vi "Get settings chain.vi"(8 "error in (no error)":errorcluster, 11 "TemplateBase in":refnum<class "PockelCell.lvclass">) -> (0 "error out":errorcluster, 1 "class name":string[](array[string]), 2 "settings":variant[](array[variant]), 3 "TemplateBase out":refnum<class "PockelCell.lvclass">)   [LabVIEW 2012, in "PockelCell.lvclass"]
doc: "Returns an array of variants containing the settings clusters of each class in the inheritance chain (lowest child class first), together with an array of all class names in the inheritance chain.\n\nFor classes without settings cluster, the settings chain contains empty variants."
uses:
  PockelCell.lvclass
  <vilib>/Distrio/Murmex/Murmex/Murmex.lvclass
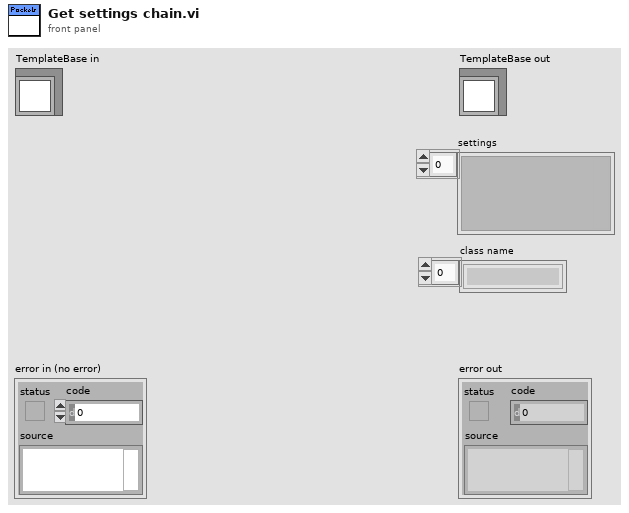
[diagram p1: front panel]
types:
  T1 = typedef "PockelCell.lvclass/settings_cluster.ctl" = cluster{"Samples per cycle":i32, "Number of cycles":i32, "Duty cycle (%)":dbl, "Analog Voltage\n":T2}
  T2 = typedef "PockelCell.lvclass/laser line PC.ctl" = dbl
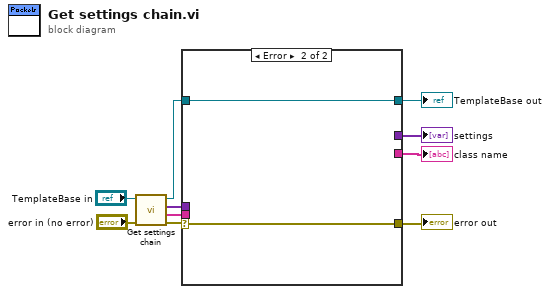
[diagram p0: block diagram]
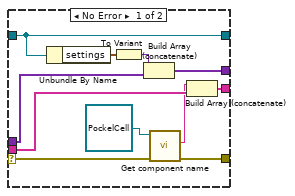
[diagram p2: hidden frame]
diagram:
  n1 = call-parent "Get settings chain.vi"("error in (no error)"="error in (no error)", "MurmexBase in"="TemplateBase in") -> ("error out"=w8:errorcluster, "class name"=w3:string[], "settings"=w4:variant[], "MurmexBase out"=w6:refnum<class "PockelCell.lvclass">)  [unwired: 6 in]
  n2 = case shown="Error" w8 {
    selector: w8 -> [w21 w22]
    tunnel: [w20 w22] -> w7
    tunnel: w6 -> [w16 w23]
    tunnel: [w16 w23] -> w5
    tunnel: w4 -> [w15 _]
    tunnel: w3 -> [w14 _]
    tunnel: [w13 _] -> w2
    tunnel: [w11 _] -> w1
    frame No Error {
      n3 = Unbundle By Name(w16) -> ("settings"=w17:T1)
      n4 = To Variant(anything=w17) -> (Variant=w18:variant)
      n5 = Build Array (concatenate)(w18, w15) -> (w13:variant[])
      n6 = call "Get component name.vi"("error in (no error)"=w21, "Murmex in"=refnum<class "PockelCell.lvclass"> refnum ("PockelsCell")) -> ("error out"=w20:errorcluster, "component name"=w12:string)  [unwired: 7 in, 1 out]
      n7 = Build Array (concatenate)(w12, w14) -> (w11:string[])
    }
    frame Error {
    }
  }
  "error out" <- w7
  "TemplateBase out" <- w5
  "settings" <- w2
  "class name" <- w1
